vi "general globals.vi"() -> ()   [LabVIEW 2014]
panel:
  out "LED Value":bool
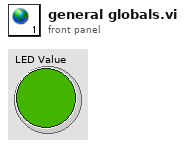
[diagram p1: front panel]
diagram:
